vi "Startup (Receive type).vi"(8 "error in (no error)":errorcluster, 11 "Startup Message":refnum<class "MSG.lvclass">) -> (0 "error out":errorcluster, 2 "Command Messenger out":refnum<class "MGR (Receive type).lvclass">, 3 "Starup Message":refnum<class "MSG.lvclass">)   [LabVIEW 2011, in "Messenging.lvlib" / "Parallel Process.lvclass"]
uses:
  Parallel Process.lvclass
  Interprocess Messenger/TextVarientMessage/MSG.lvclass
  Interprocess Messenger/TextVarientMessage/Reply (message).vi
  Interprocess Messenger/QueueMessenger/QueueMessenger.lvclass
  Interprocess Messenger/TextVarientMessage/Write (no data).vi
  Interprocess Messenger/Receiver/MGR (Receive type).lvclass
  Interprocess Messenger/TextVarientMessage/Extract Object (static).vi
  Interprocess Messenger/TextVarientMessage/Write VarMessage.vi
  Interprocess Messenger/VarMessage/VarMessage.lvclass
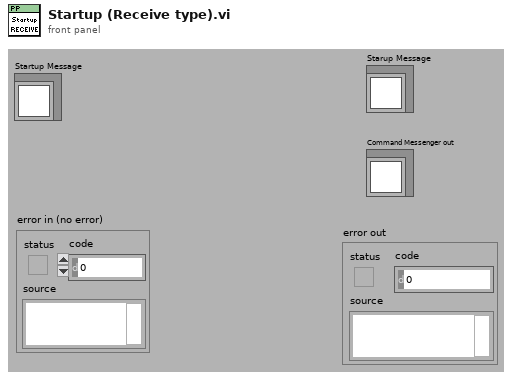
[diagram p1: front panel]
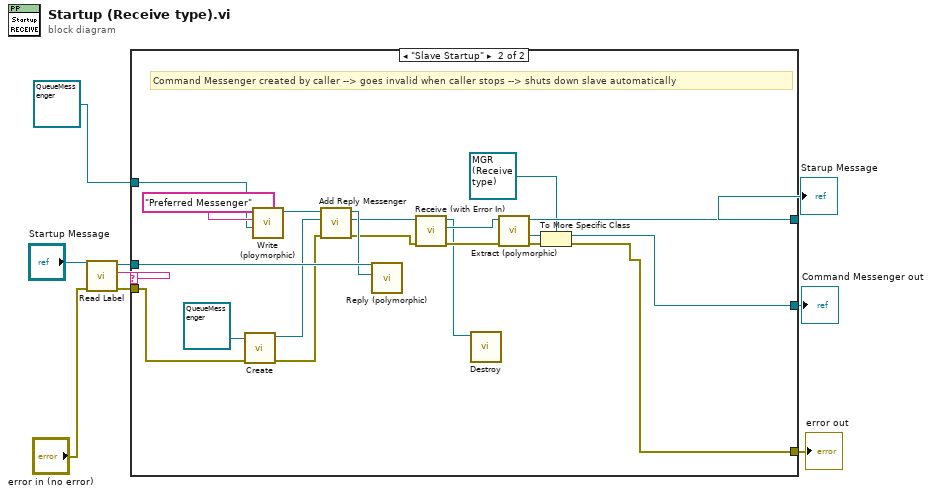
[diagram p0: block diagram]
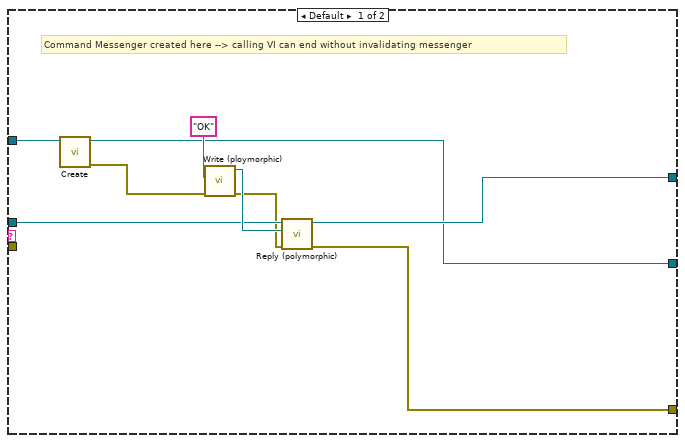
[diagram p2: hidden frame]
diagram:
  n1 = call-dynamic "Read Label.vi"("error in (no error)"="error in (no error)", "Message"="Startup Message") -> ("error out"=w4:errorcluster, "Label"=w8:string, "Message"=w7:refnum<class "MSG.lvclass">)  [unwired: 7 out]
  n2 = case shown="\"Slave Startup\"" w8 {
    tunnel: w7 -> [w15 w36]
    tunnel: refnum<class "QueueMessenger.lvclass"> refnum ("Messenging.lvlib:QueueMessenger.lvclass") -> [w18 w32]
    tunnel: [w14 w30] -> w6
    tunnel: [w13 w20] -> w1
    tunnel: w4 -> [_ w22]
    tunnel: [w10 w21] -> w3
    frame Default {
      # "Command Messenger created here --> calling VI can end without invalidating messenger"
      n3 = call-dynamic "Create.vi"("QueueMessenger in"=w18) -> ("error out"=w12:errorcluster, "QueueMessenger out"=w13:refnum<class "QueueMessenger.lvclass">)  [unwired: 1 in, 8 out]
      n4 = call-poly "Write (ploymorphic).vi"("error in (no error)"=w12, "Label"="OK") -> ("error out"=w11:errorcluster, "Message"=w16:refnum<class "MSG.lvclass">)  [unwired: 8 out]
      n5 = call-poly "Reply (polymorphic).vi"("error in (no error)"=w11, "Reply"=w16, "Message to Reply to"=w15) -> ("error out"=w10:errorcluster, "Message"=w14:refnum<class "MSG.lvclass">)  [unwired: 7 out]
    }
    frame "Slave Startup" {
      # "Command Messenger created by caller --> goes invalid when caller stops --> shuts down slave automatically"
      n6 = call-dynamic "Create.vi"("error in (no error)"=w22, "QueueMessenger in"=refnum<class "QueueMessenger.lvclass"> refnum ("QueueMessenger.lvclass")) -> ("error out"=w24:errorcluster, "QueueMessenger out"=w26:refnum<class "QueueMessenger.lvclass">)  [unwired: 8 out]
      n7 = call-poly "Write (ploymorphic).vi"("Varient"=w32, "Label"="Preferred Messenger") -> ("Message"=w37:refnum<class "VarMessage.lvclass">)  [unwired: 1 in, 8 out]
      n8 = call "Add Reply Messenger.vi"("error in (no error)"=w24, "Reply to..."=w26, "Message"=w37) -> ("error out"=w23:errorcluster, "Reply to..."=w34:refnum<class "QueueMessenger.lvclass">, "Message"=w35:refnum<class "VarMessage.lvclass">)  [unwired: 6 out]
      n9 = call-poly "Reply (polymorphic).vi"("Reply"=w35, "Message to Reply to"=w36) -> ()  [unwired: 1 in, 9 out]
      n10 = call-dynamic "Receive (with Error In).vi"("error in (no error)"=w23, "MGR in"=w34) -> ("error out"=w31:errorcluster, "Message"=w33:refnum<class "MSG.lvclass">, "MGR out"=w25:refnum<class "QueueMessenger.lvclass">)  [unwired: 1 in, 6 out]
      n11 = call-dynamic "Destroy.vi"("QueueMessenger in"=w25) -> ()  [unwired: 1 in, 10 out]
      n12 = call-poly "Extract (polymorphic).vi"("error in (no error)"=w31, "ObjMessage in"=w33) -> ("error out"=w29:errorcluster, "Object"=w28:refnum<class>, "ObjMessage out"=w30:refnum<class "MSG.lvclass">)  [unwired: 7 out]
      n13 = To More Specific Class(target class=refnum<class "MGR (Receive type).lvclass"> refnum ("Command Messenger out"), reference=w28, error in=w29) -> (specific class reference=w20:refnum<class "MGR (Receive type).lvclass">, error out=w21:errorcluster)
    }
  }
  "Command Messenger out" <- w1
  "Starup Message" <- w6
  "error out" <- w3
